vi "_Open Simulation File.vi"(6 "AcqMethod":T1[](array[typedef]) {"ScanType" format="%#.6g"; "Mass Range"."Res" items=["High/High", "Medium/Medium", "Low/Low", "High/Medium", "High/Low", "Medium/High", "Medium/Low", "Low/High", "Low/Medium"]}, 8 "ErrorIn":errorcluster, 11 "FileRefIn":refnum<file>) -> (0 "ErrorOut":errorcluster, 1 "Mass":dbl[](array[numeric]), 2 "Index Array":i64[][](array[numeric]), 3 "FileRefOut":refnum<file>, 4 "TIC":u32[](array[numeric]), 5 "Steps":i32, 7 "Version":i32)   [LabVIEW 2015]
uses:
  Type/_XML Expt.ctl
  Type/_XML Lens.ctl
  Type/_Mass Range Property.ctl
  Type/_Mass Range Parameters.ctl
  Type/_RT Res Type.ctl
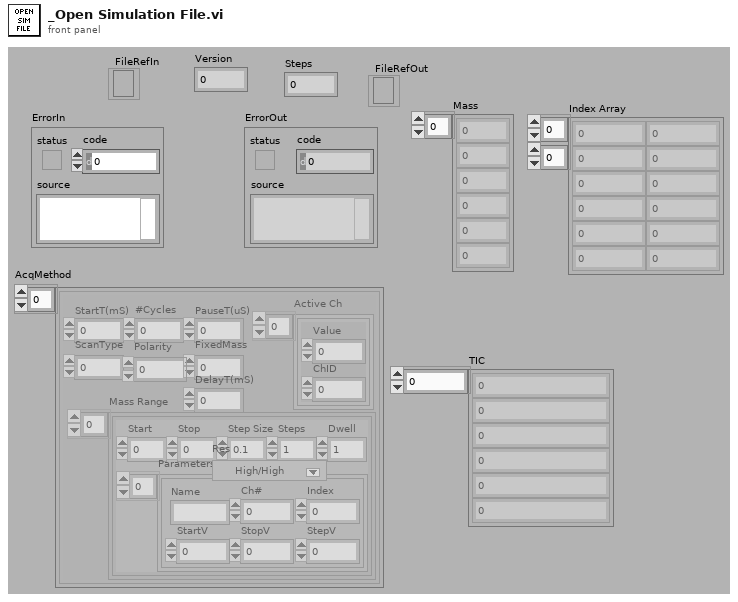
[diagram p1: front panel]
types:
  T1 = typedef "_XML Expt.ctl" = cluster{"StartT(mS)":i32, "#Cycles":i32, "PauseT(uS)":i32, "ScanType":i32, "Polarity":u8, "FixedMass":dbl, "DelayT(mS)":i32, "Active Ch":T2[], "Mass Range":T3[]}
  T2 = typedef "_XML Lens.ctl" = cluster{"Value":dbl, "ChID":u8}
  T3 = typedef "_Mass Range Property.ctl" = cluster{"Start":dbl, "Stop":dbl, "Step Size":dbl, "Steps":i32, "Dwell":dbl, "Parameters":T4[], "Res":T5}
  T4 = typedef "_Mass Range Parameters.ctl" = cluster{"Name":string, "Ch#":u8, "StartV":dbl, "StopV":dbl, "StepV":dbl, "Index":u8}
  T5 = typedef "_RT Res Type.ctl" = u16
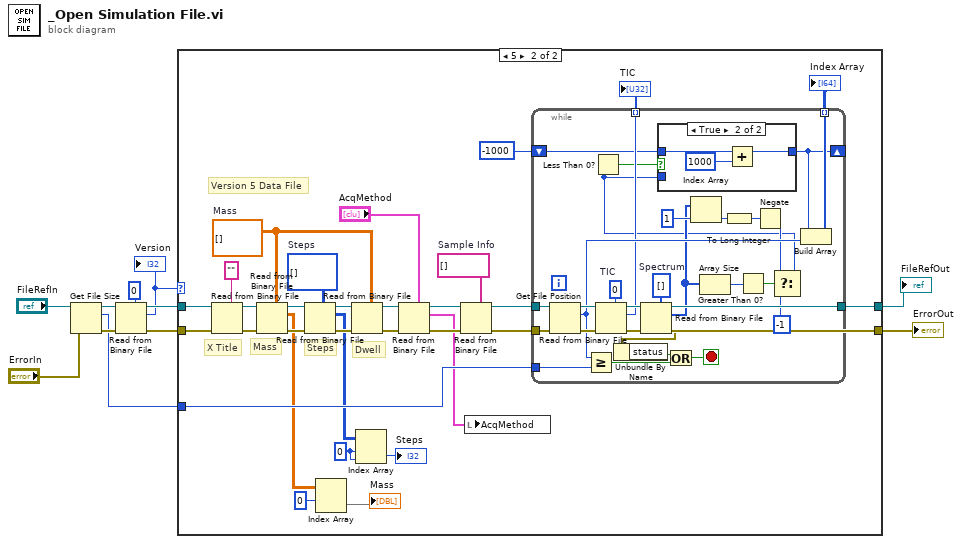
[diagram p0: block diagram]
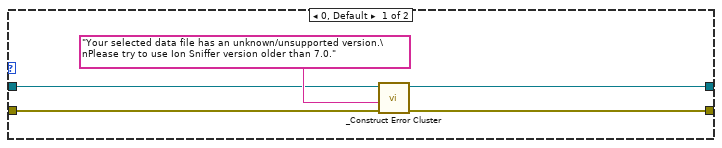
[diagram p2: hidden frame]
diagram:
  n1 = Get File Size ("EOF")(file="FileRefIn", error in="ErrorIn") -> (refnum out=w10:refnum<file>, size (in bytes)=w6:i64, 0:w9:errorcluster)
  n2 = Read from Binary File(5:0 ("pos offset (0)"), 8:w9, 11:w10) -> (0:w7:errorcluster, 2:w5:i32, 3:w8:refnum<file>)  [unwired: 4 out]
  "Version" <- w5
  n3 = case shown="5" w5 {
    tunnel: w7 -> [w15 w44]
    tunnel: w8 -> [w12 w43]
    tunnel: [w13 w17] -> w4
    tunnel: w6 -> [_ w36]
    tunnel: [w12 w16] -> w1
    frame 0, Default {
      n4 = call "_Construct Error Cluster.vi"("error in"=w15, "reason"="Your selected data file has an unknown/unsupported version.\nPlease try to use Ion Sniffer version older than 7.0.") -> ("error out"=w13:errorcluster)  [unwired: 2 in, 3 out]
    }
    frame 5 {
      w25 = 0 ("index (row)")
      w28 = dbl[][] []  # Mass
      w29 = i32[][] []  # Steps
      w32 = string[] []  # Sample Info
      # "Steps"
      # "X Title"
      # "Dwell"
      # "Mass"
      # "Version 5 Data File"
      n5 = Read from Binary File(5:"", 8:w44, 11:w43) -> (0:w46:errorcluster, 3:w42:refnum<file>)  [unwired: 5 out]
      n6 = Read from Binary File(5:w28, 8:w46, 11:w42) -> (0:w45:errorcluster, 2:w23:dbl[][], 3:w41:refnum<file>)  [unwired: 4 out]
      n7 = Read from Binary File(5:w29, 8:w45, 11:w41) -> (0:w38:errorcluster, 2:w26:i32[][], 3:w39:refnum<file>)  [unwired: 4 out]
      n8 = Index Array(array=w23, index (row)=0) -> (element=→"Mass":dbl[])  [unwired: 1 in]
      n9 = Read from Binary File(5:w28, 8:w38, 11:w39) -> (0:w40:errorcluster, 3:w37:refnum<file>)  [unwired: 5 out]
      n10 = Index Array(array=w26, index (row)=w25, index (col)=w25) -> (element=→"Steps":i32)
      n11 = Read from Binary File(5:"AcqMethod", 8:w40, 11:w37) -> (0:w33:errorcluster, 2:w30:T1[], 3:w35:refnum<file>)  [unwired: 4 out]
      n12 = Read from Binary File(5:w32, 8:w33, 11:w35) -> (0:w17:errorcluster, 3:w34:refnum<file>)  [unwired: 5 out]
      n13 = local write "AcqMethod"(w30) -> ()
      n14 = while {
        tunnel: w34 -> [w75]
        tunnel: w17 -> [w51]
        tunnel: [w73] -> w16
        tunnel: w36 -> [w72]
        tunnel: [w58] -> w18 mode=indexing
        tunnel: [w52] -> w19 mode=indexing
        shift-right: [w47] -> _
        shift-left: -1000 -> [w49]
        stop <- w69 stop-if-true
        w64 = u32 0  # TIC
        w74 = u32[] []  # Spectrum
        n15 = Get File Position(4:w51, 7:w75) -> (0:w65:errorcluster, 2:w59:i64, 3:w67:refnum<file>)
        n16 = Greater Or Equal?(x=w59, y=w72) -> (x >= y?=w70:bool)
        n17 = Read from Binary File(5:w64, 8:w65, 11:w67) -> (0:w68:errorcluster, 2:w52:u32, 3:w66:refnum<file>)  [unwired: 4 out]
        n18 = Read from Binary File(5:w74, 8:w68, 11:w66) -> (0:w63:errorcluster, 2:w57:u32[], 3:w73:refnum<file>)  [unwired: 4 out]
        n19 = Unbundle By Name(w63) -> ("status"=w71:bool)
        n20 = Or(x=w71, y=w70) -> (x .or. y?=w69:bool)
        n21 = Index Array(array=w57, index=1) -> (element=w61:u32)
        n22 = Array Size(array=w57) -> (size(s)=w56:i32)
        n23 = To Long Integer(number=w61) -> (32bit integer=w62:i32)
        n24 = Greater Than 0?(x=w56) -> (x > 0?=w55:bool)
        n25 = Negate(x=w62) -> (-x=w54:i32)
        n26 = Select(t=w54, s=w55, f=-1) -> (s? t:f=w48:i32)
        n27 = Less Than 0?(x=w48) -> (x < 0?=w50:bool)
        n28 = case shown="True" w50 {
          tunnel: w49 -> [_ w79]
          tunnel: [w76 w77] -> w47
          tunnel: w48 -> [w76 _]
          frame False {
          }
          frame True {
            n29 = Add(x=w79, y=1000) -> (x+y=w77:i32)
          }
        }
        n30 = Build Array(w47, w59) -> (w58:i64[])
      }
      "Index Array" <- w18
      "TIC" <- w19
    }
  }
  "ErrorOut" <- w4
  "FileRefOut" <- w1
